vi "getWaypoints.vi"(8 "Error In":errorcluster, 11 "GenericMission in":refnum<class "GenericMission.lvclass">) -> (0 "Error Out":errorcluster, 2 "Waypoint Array":refnum<class "Waypoint.lvclass">[](array[class]), 3 "GenericMission out":refnum<class "GenericMission.lvclass">)   [LabVIEW 2012, in "GenericMission.lvclass"]
uses:
  GenericMission.lvclass
  Waypoint/Waypoint.lvclass
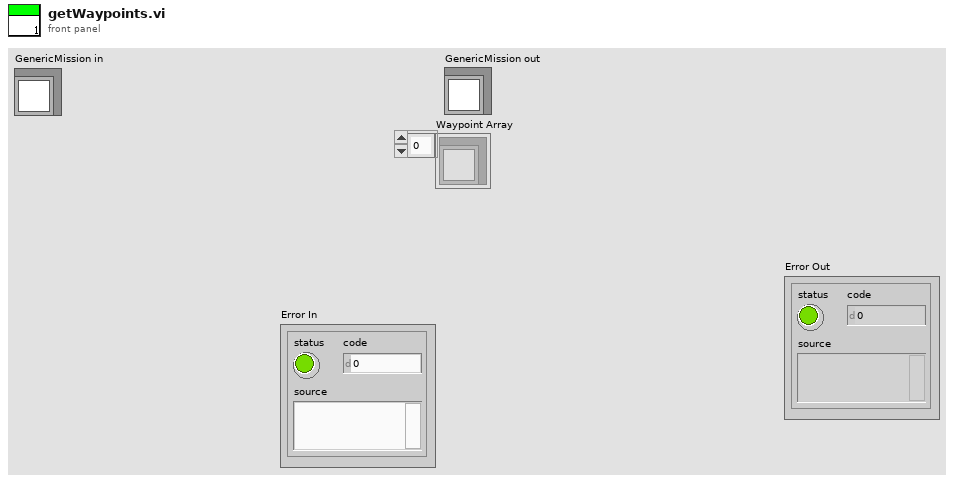
[diagram p1: front panel]
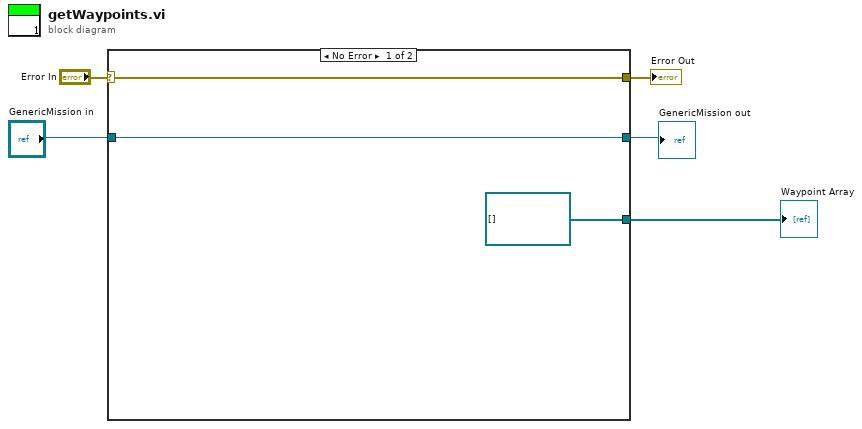
[diagram p0: block diagram]
diagram:
  n1 = case shown="No Error" "Error In" {
    selector: "Error In" -> [w7 w9]
    tunnel: [w7 w9] -> w4
    tunnel: "GenericMission in" -> [w8 w10]
    tunnel: [w8 w10] -> w3
    tunnel: [refnum<class "Waypoint.lvclass">[] [] ("Array 2") _] -> w1
    frame No Error {
    }
    frame Error {
    }
  }
  "Error Out" <- w4
  "GenericMission out" <- w3
  "Waypoint Array" <- w1
